vi "Control.vi"(9 "SensorInputData":T5, 10 "ActuatorInputs":T6, 11 "HMI to Control":T1={"RightDriveValue"=0.0, "LeftDriveValue"=0.0, "Intake Value"=0.0, "Shooter States"=enum."Shooter Off", "Collector Lift States"=enum."Collector Manual", "Shooter Hood States"=enum."Hood Close Shot", "Fire "=FALSE, "Collector Lift Manual Value"=0.0, "Shooter Hood Manual Value"=0.0, " Autolift portcullis"=FALSE, "Autoadjust CDF"=FALSE, "Hood Manual Request"=FALSE, "Collect Lift Manual Request"=FALSE, "Keep at target "=FALSE, "Hood Manual No."=0, "Collect Lift Manual No. "=0}) -> (2 "ActuatorInputs Out":T6, 3 "HMI to Control Out":T1={"RightDriveValue"=0.0, "LeftDriveValue"=0.0, "Intake Value"=0.0, "Shooter States"=enum."Shooter Off", "Collector Lift States"=enum."Collector Manual", "Shooter Hood States"=enum."Hood Close Shot", "Fire "=FALSE, "Collector Lift Manual Value"=0.0, "Shooter Hood Manual Value"=0.0, " Autolift portcullis"=FALSE, "Autoadjust CDF"=FALSE, "Hood Manual Request"=FALSE, "Collect Lift Manual Request"=FALSE, "Keep at target "=FALSE, "Hood Manual No."=0, "Collect Lift Manual No. "=0})   [LabVIEW 2015]
uses:
  Typedefs/HMI_to_Control.ctl
  Typedefs/Shooter States.ctl
  Typedefs/CollectorLiftStates.ctl
  Typedefs/Hood States.ctl
  Typedefs/ActuatorInputs.ctl
  Typedefs/SensorInputData.ctl
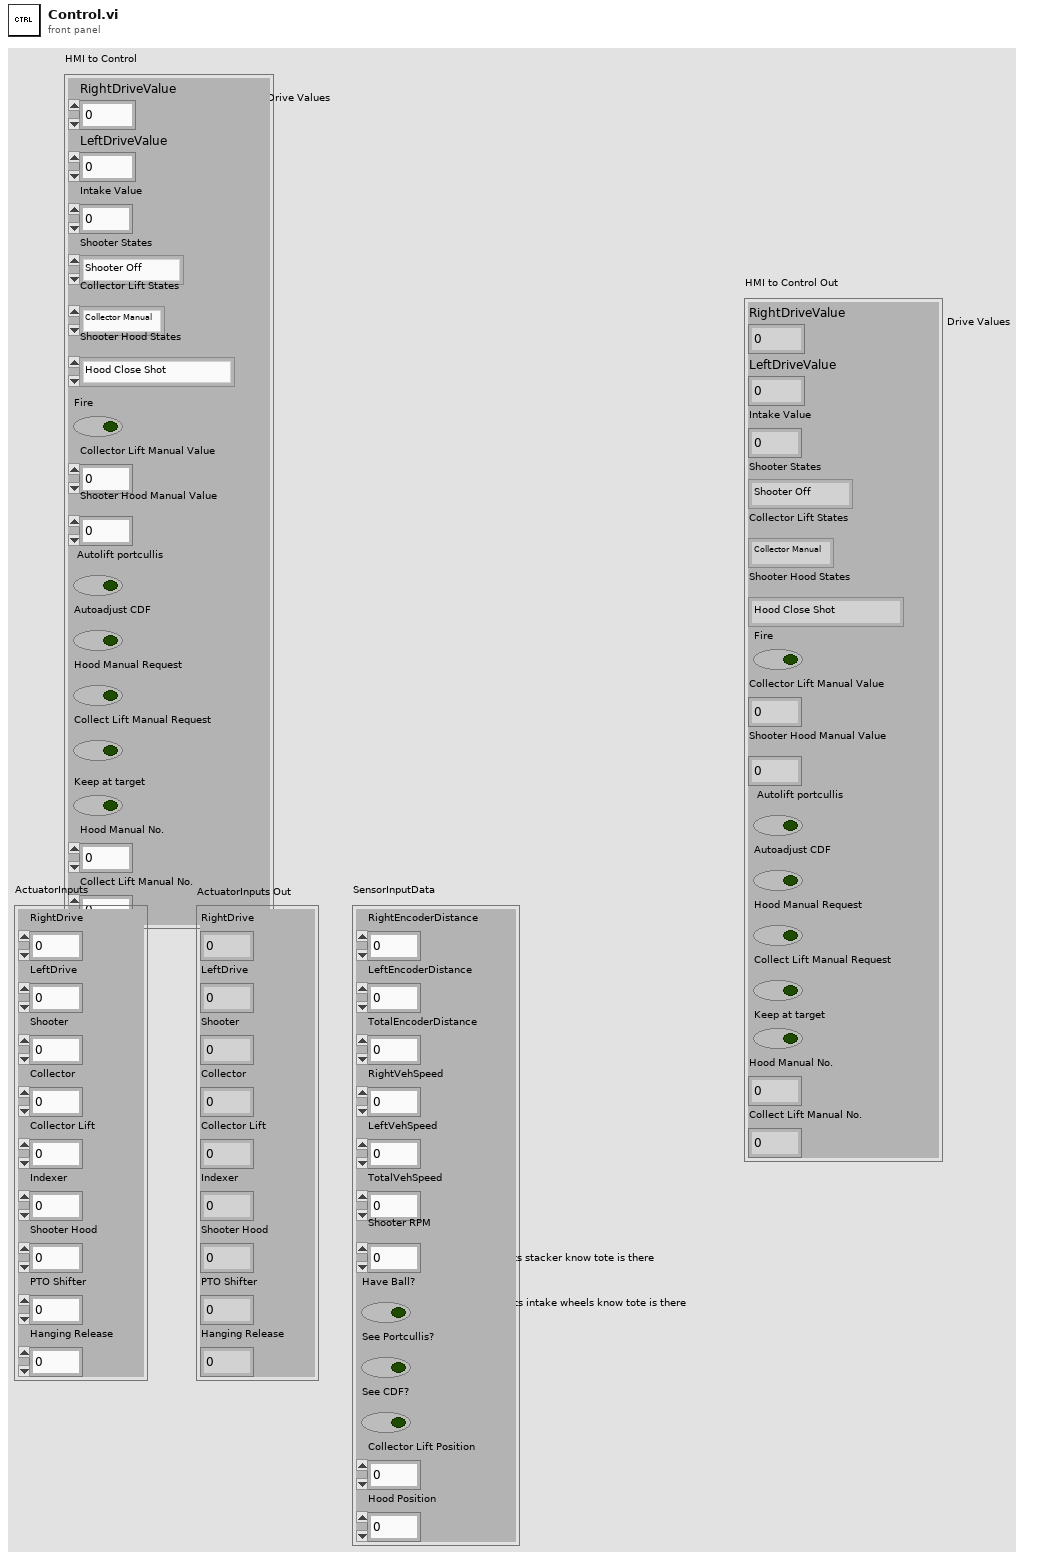
[diagram p1: front panel]
types:
  T1 = typedef "HMI_to_Control.ctl" = cluster{"RightDriveValue":dbl, "LeftDriveValue":dbl, "Intake Value":dbl, "Shooter States":T2, "Collector Lift States":T3, "Shooter Hood States":T4, "Fire ":bool, "Collector Lift Manual Value":dbl, "Shooter Hood Manual Value":dbl, " Autolift portcullis":bool, "Autoadjust CDF":bool, "Hood Manual Request":bool, "Collect Lift Manual Request":bool, "Keep at target ":bool, "Hood Manual No.":i8, "Collect Lift Manual No. ":i8}
  T2 = typedef "Shooter States.ctl" = enum16{"Shooter Off", "Shooter Far", "Shooter Close", "Shooter Intermediate", "Shooter Spy"}
  T3 = typedef "CollectorLiftStates.ctl" = enum16{"Collector Manual", "Stow", "Collect Position", "Spit Position", "Portcullis Set Up", "Portcullis Lift Up", "CDF Set Up", "Push CDF Down"}
  T4 = typedef "Hood States.ctl" = enum16{"Hood Manual ", "Hood Close Shot", "Hood Far Shot", "Hood Spy Shot", "Hood Intermediate"}
  T5 = typedef "SensorInputData.ctl" = cluster{"RightEncoderDistance":dbl, "LeftEncoderDistance":dbl, "TotalEncoderDistance":dbl, "RightVehSpeed":dbl, "LeftVehSpeed":dbl, "TotalVehSpeed":dbl, "Shooter RPM":dbl, "Have Ball?":bool, "See Portcullis?":bool, "See CDF?":bool, "Collector Lift Position":dbl, "Hood Position":dbl}
  T6 = typedef "ActuatorInputs.ctl" = cluster{"RightDrive":dbl, "LeftDrive":dbl, "Shooter":dbl, "Collector":dbl, "Collector Lift":dbl, "Indexer":dbl, "Shooter Hood":dbl, "PTO Shifter":dbl, "Hanging Release":dbl}
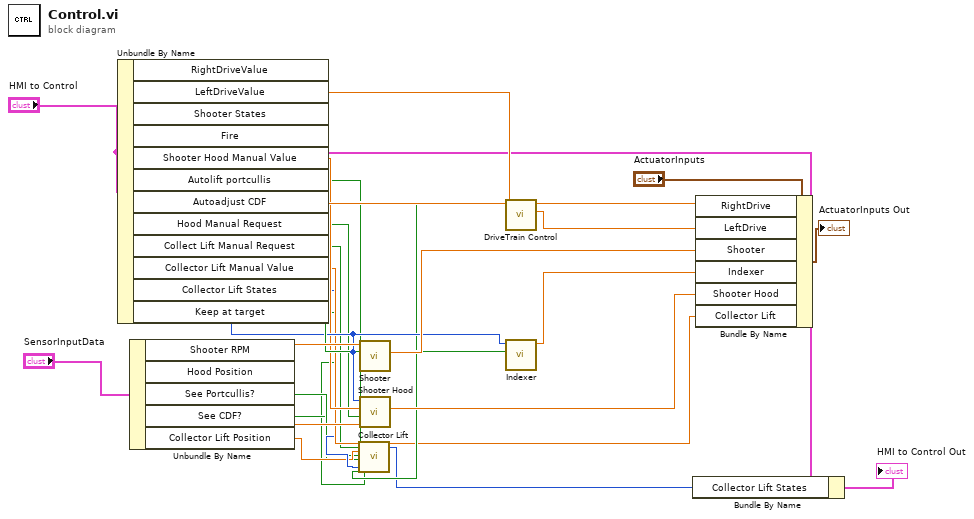
[diagram p0: block diagram]
diagram:
  n1 = Unbundle By Name("HMI to Control") -> ("RightDriveValue"=w27:dbl, "LeftDriveValue"=w26:dbl, "Shooter States"=w18:T2, "Fire"=w20:bool, "Shooter Hood Manual Value"=w17:dbl, "Autolift portcullis"=w10:bool, "Autoadjust CDF"=w11:bool, "Hood Manual Request"=w14:bool, "Collect Lift Manual Request"=w12:bool, "Collector Lift Manual Value"=w13:dbl, "Collector Lift States"=w9:T3, "Keep at target"=w4:bool)
  n2 = Unbundle By Name("SensorInputData") -> ("Shooter RPM"=w21:dbl, "Hood Position"=w16:dbl, "See Portcullis?"=w7:bool, "See CDF?"=w6:bool, "Collector Lift Position"=w8:dbl)
  n3 = call "Collector Lift.vi"("Collector Lift Man. Value"=w13, "Collector Lift Man.  Request?"=w12, "Collector Lift Postion"=w8, "See Portcullis?"=w7, "See CDF?"=w6, "AutoLift Portcullis?"=w10, "Collector Lift States"=w9, "AutoAdjust CDF?"=w11, "Keep at Target?"=w4) -> ("Collector Lift Output"=w5:dbl, "Collector Lift State Out"=w1:T3)  [unwired: 17 in]
  n4 = call "Shooter.vi"("Shooter States"=w18, "Shooter RPM"=w21) -> ("Shooter Output"=w22:dbl)  [unwired: 8 in, 1 out]
  n5 = call "Shooter Hood.vi"("Hood Position"=w16, "Hood Man. Request?"=w14, "Hood Manual Value"=w17, "Shooter States"=w18) -> ("Shooter Hood Output"=w15:dbl)  [unwired: 6 in, 1 out]
  n6 = call "DriveTrain Control.vi"("Left Drive In"=w26, "Right Drive In"=w27) -> ("Left Drive Out"=w24:dbl, "Right Drive Out"=w25:dbl)  [unwired: 8 in]
  n7 = call "Indexer.vi"("Fire"=w20, "Shooter States"=w18) -> ("Indexer Value"=w19:dbl)  [unwired: 9 in]
  n8 = Bundle By Name(cluster="HMI to Control", "Collector Lift States"=w1) -> (→"HMI to Control Out":T1)
  n9 = Bundle By Name(cluster="ActuatorInputs", "RightDrive"=w25, "LeftDrive"=w24, "Shooter"=w22, "Indexer"=w19, "Shooter Hood"=w15, "Collector Lift"=w5) -> (→"ActuatorInputs Out":T6)
